vi "Delete_file.vi"(8 "error in":errorcluster, 11 "Filename (ini)":string="Config_Ver_2\\state_library") -> (0 "error out":errorcluster)   [LabVIEW 2021]
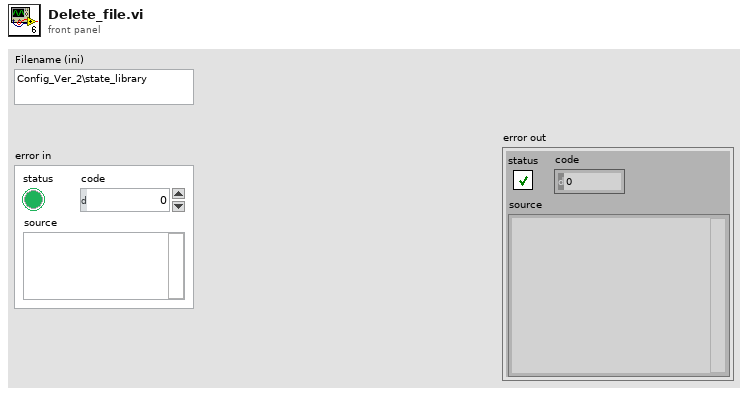
[diagram p1: front panel]
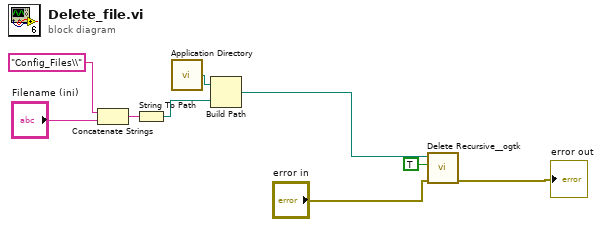
[diagram p0: block diagram]
diagram:
  n1 = Concatenate Strings("Config_Files\\" ("string"), "Filename (ini)") -> (w5:string)
  n2 = String To Path(string=w5) -> (path=w6:path)
  n3 = call <vilib>:"Application Directory.vi"() -> ("Application Directory"=w8:path)
  n4 = Build Path(base path=w8, name or relative path=w6) -> (appended path=w4:path)
  n5 = call <userlib>:"Delete Recursive__ogtk.vi"("error in (no error)"="error in", "Recursive? (FALSE)"=TRUE, "Path"=w4) -> ("error out"=→"error out":errorcluster)  [unwired: 7 in, 1 out]
